vi "Periodic Tasks.vi"(8 "error in":errorcluster) -> ()   [LabVIEW 2019]
doc: "This VI runs in parallel to other tasks. It can contain as many user-defined periodic loops as you need. These can carry out PID or other sorts of timed response."
uses:
  <vilib>/Rock Robotics/SystemInterfaces/i2clib/i2c_bus.ctl
  <vilib>/Rock Robotics/Network Tables/NT Write Number.vi
  <vilib>/Rock Robotics/Network Tables/NT Write String.vi
panel:
  in  "Blue Calibration":cluster{"R":dbl, "G":dbl, "B":dbl}={"R"=65.0, "G"=118.0, "B"=67.0}
  in  "Green Calibration":cluster{"R":dbl, "G":dbl, "B":dbl}={"R"=69.0, "G"=124.0, "B"=59.0}
  in  "Red Calibration":cluster{"R":dbl, "G":dbl, "B":dbl}={"R"=98.0, "G"=107.0, "B"=47.0}
  in  "Yellow Calibration":cluster{"R":dbl, "G":dbl, "B":dbl}={"R"=89.0, "G"=122.0, "B"=42.0}
  in  "I2C Bus":T1
  out "Color":u32(colorbox)
  out "Proximity":u16(graph)
  out "error out":errorcluster
  out "Measured Color":cluster{"R":dbl, "G":dbl, "B":dbl}
  out "Match Confidence":dbl
  out "Matched Color Name":string
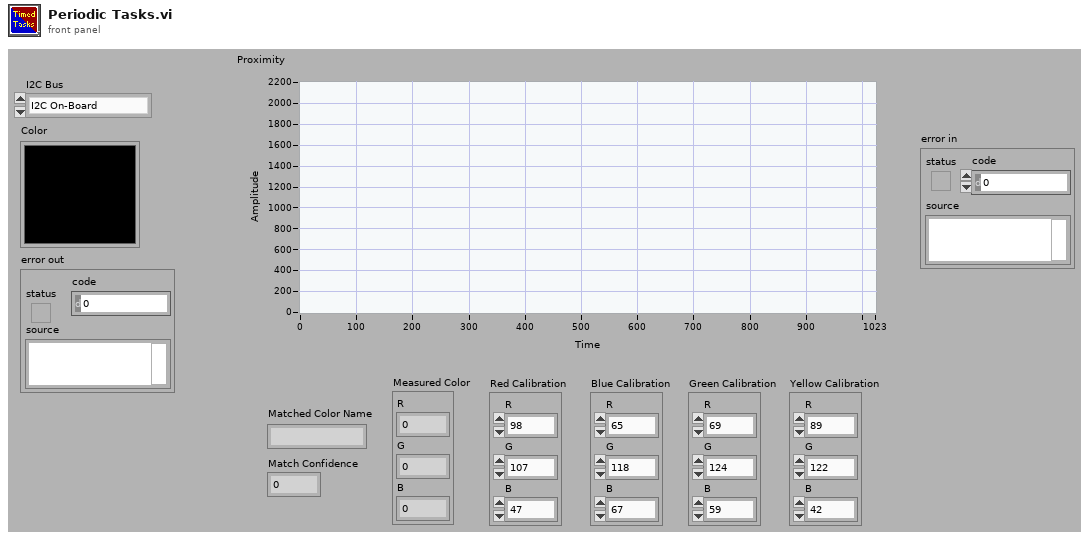
[diagram p1: front panel]
types:
  T1 = typedef "i2c_bus.ctl" = enum16{"I2C On-Board", "I2C MXP", "Invalid"}
  T2 = typedef "Color Sensor V3 DevRef.ctl" = cluster{"I2CDevRef":T3}
  T3 = typedef "WPI_I2CDevRef.ctl" = cluster{"DevStatus":errorcluster, "Device Address":u8, "Handle":i32, "I2C Bus":T1}
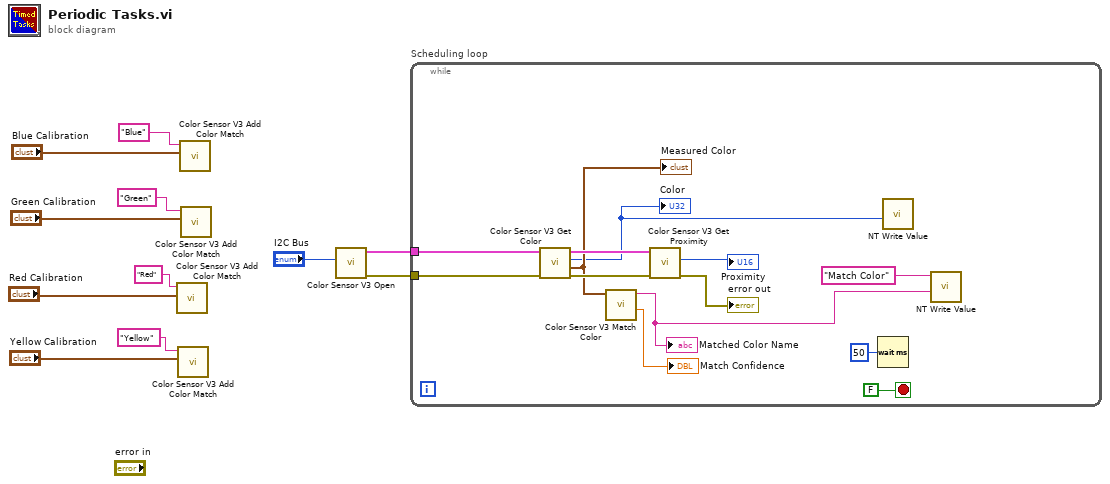
[diagram p0: block diagram]
diagram:
  n1 = call <vilib>:"Color Sensor V3 Add Color Match.vi"("Color"="Red Calibration", "Name"="Red") -> ()  [unwired: 10 in]
  n2 = call <vilib>:"Color Sensor V3 Add Color Match.vi"("Color"="Yellow Calibration", "Name"="Yellow") -> ()  [unwired: 10 in]
  n3 = call <vilib>:"Color Sensor V3 Add Color Match.vi"("Color"="Blue Calibration", "Name"="Blue") -> ()  [unwired: 10 in]
  n4 = call <vilib>:"Color Sensor V3 Add Color Match.vi"("Color"="Green Calibration", "Name"="Green") -> ()  [unwired: 10 in]
  n5 = call <vilib>:"Color Sensor V3 Open.vi"("I2C Bus"="I2C Bus") -> ("error out"=w9:errorcluster, "ColorSensorDevRef"=w10:T2)  [unwired: 9 in]
  n6 = while "Scheduling loop" {
    tunnel: w10 -> [w19]
    tunnel: w9 -> [w18]
    stop <- FALSE stop-if-true
    n7 = call <vilib>:"Color Sensor V3 Get Color.vi"("error in (no error)"=w18, "ColorSensorDevRef"=w19) -> ("error out"=w23:errorcluster, "Normalized Color"=w17:cluster{"R":dbl, "G":dbl, "B":dbl}, "Color"=w12:u32, "ColorSensorDevRef out"=w22:T2)  [unwired: 6 in]
    "Color" <- w12
    "Measured Color" <- w17
    n8 = call <vilib>:"Color Sensor V3 Match Color.vi"("Measured Color"=w17) -> ("Confidence"=→"Match Confidence":dbl, "Matched Color Name"=w14:string)  [unwired: 8 in, 1 out]
    "Matched Color Name" <- w14
    n9 = call <vilib>:"Color Sensor V3 Get Proximity.vi"("error in (no error)"=w23, "ColorSensorDevRef"=w22) -> ("error out"=→"error out":errorcluster, "Proximity"=→"Proximity":u16)  [unwired: 7 in, 1 out]
    n10 = Wait (ms)(milliseconds to wait=u32 50) -> ()  [unwired: 1 out]
    n11 = call-poly <vilib>:"NT Write Value.vi"("Numeric"=w12) -> ()  [unwired: 10 in, 1 out]
    n12 = call-poly <vilib>:"NT Write Value.vi"("String"=w14, "Name"="Match Color") -> ()  [unwired: 9 in, 1 out]
  }
